vi "getBroadcastAdresses.vi"(4 "error in (no error)":errorcluster) -> (0 "error out":errorcluster, 1 "broadcast addresses":u32[](array[numeric]), 2 "IP addresses":u32[](array[numeric]), 3 "number of IPs":i32)   [LabVIEW 2013]
uses:
  IPConnections.dll
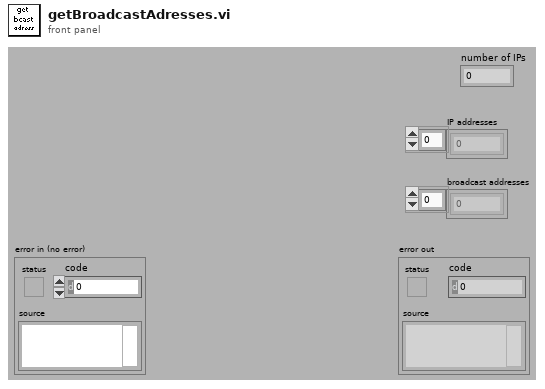
[diagram p1: front panel]
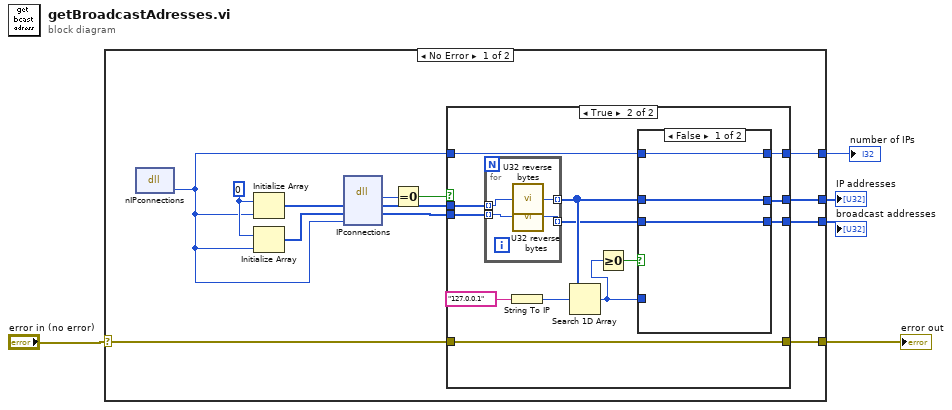
[diagram p0: block diagram]
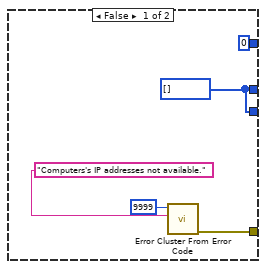
[diagram p2: hidden frame]
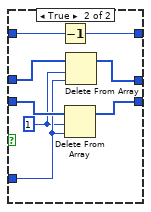
[diagram p3: hidden frame]
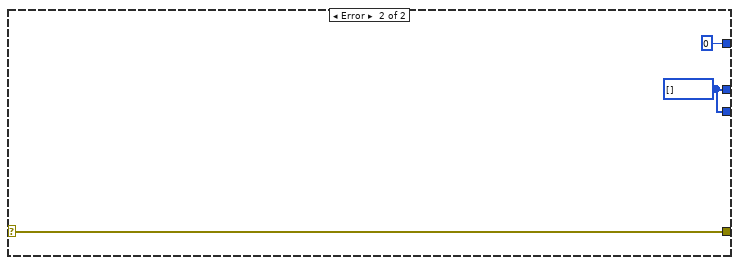
[diagram p4: hidden frame]
diagram:
  n1 = case shown="No Error" "error in (no error)" {
    selector: "error in (no error)" -> [w8 w54]
    tunnel: [w13 w52] -> w2
    tunnel: [w12 w52] -> w1
    tunnel: [w9 w54] -> w4
    tunnel: [w6 0] -> w3
    frame No Error {
      w17 = u32 0
      n2 = dll-call lib="L:/cwthz/cwterahertz/Examples/DeCof SubVI Library/IPconnections/IPconnections.dll" fn="nIPconnections"() -> (w7:i32)  [unwired: 3 in, 2 out]
      n3 = Initialize Array(w17, w7) -> (w18:u32[])
      n4 = Initialize Array(w17, w7) -> (w16:u32[])
      n5 = dll-call lib="L:/cwthz/cwterahertz/Examples/DeCof SubVI Library/IPconnections/IPconnections.dll" fn="IPconnections"("addresses"=w18, "broadcasts"=w16, "n"=w7) -> (w11:i32, "addresses"=w15:u32[], "broadcasts"=w14:u32[])  [unwired: 4 in, 2 out]
      n6 = Equal To 0?(x=w11) -> (x = 0?=w10:bool)
      n7 = case shown="True" w10 {
        tunnel: w15 -> [_ w36]
        tunnel: w14 -> [_ w35]
        tunnel: [w19 w29] -> w13
        tunnel: [w19 w27] -> w12
        tunnel: [w22 w34] -> w9
        tunnel: w8 -> [_ w34]
        tunnel: w7 -> [_ w33]
        tunnel: [0 w26] -> w6
        frame False {
          w19 = u32[] []
          n8 = call <vilib>:"Error Cluster From Error Code.vi"("error message (\"\")"="Computers's IP addresses not available." ("error message (\"\")"), "error code (0)"=9999) -> ("error out"=w22:errorcluster)  [unwired: 7 in]
        }
        frame True {
          n9 = for {
            tunnel: w36 -> [w51] mode=indexing
            tunnel: w35 -> [w50] mode=indexing
            tunnel: [w49] -> w30 mode=indexing
            tunnel: [w48] -> w28 mode=indexing
            n10 = call "U32 reverse bytes.vi"("U32 in"=w51) -> ("U32 out"=w49:u32)
            n11 = call "U32 reverse bytes.vi"("U32 in"=w50) -> ("U32 out"=w48:u32)
          }
          n12 = String To IP(1:"127.0.0.1" ("name")) -> (0:w31:u32)
          n13 = Search 1D Array(1D array=w30, element=w31) -> (index of element=w25:i32)  [unwired: 1 in]
          n14 = Greater Or Equal To 0?(x=w25) -> (x >= 0?=w24:bool)
          n15 = case shown="False" w24 {
            tunnel: w33 -> [w39 w47]
            tunnel: w30 -> [w38 w46]
            tunnel: [w38 w45] -> w29
            tunnel: w28 -> [w37 w44]
            tunnel: [w37 w43] -> w27
            tunnel: w25 -> [_ w42]
            tunnel: [w39 w40] -> w26
            frame False {
            }
            frame True {
              w41 = 1
              n16 = Decrement(x=w47) -> (x-1=w40:i32)
              n17 = Delete From Array(array=w44, length=w41, index=w42) -> (array with subset deleted=w43:u32[])  [unwired: 1 out]
              n18 = Delete From Array(array=w46, length=w41, index=w42) -> (array with subset deleted=w45:u32[])  [unwired: 1 out]
            }
          }
        }
      }
    }
    frame Error {
      w52 = u32[] []
    }
  }
  "error out" <- w4
  "number of IPs" <- w3
  "IP addresses" <- w2
  "broadcast addresses" <- w1
